vi "KundtsTube.vi"() -> ()   [LabVIEW 2015]
uses:
  <vilib>/imath/engines/lvmath2/RunTimeEngine/Managers/WorkSpace/UID Generator.vi
  <vilib>/imath/engines/lvmath2/RunTimeEngine/RunTimeType/NIMS_RunTimeType_From StrictType (excl LVString).vi
  <instcachedir>/0/NIMS_RunTimeType_From StrictType (excl LVString)_EB1C38A9BC5048DA9ABDA8F781E54D21.lvgen/NIMS_RunTimeType_From StrictType (excl LVString)_EB1C38A9BC5048DA9ABDA8F781E54D21_000.vi
  <vilib>/imath/engines/lvmath2/RunTimeEngine/LocalVariableDefStatement/MC_LocalVariableDefStatement_Display.vi
  <vilib>/imath/engines/lvmath2/RunTimeEngine/Managers/SymbolTable/Clear UID.vi
  <vilib>/imath/engines/lvmath2/RunTimeEngine/NodeEndStatement/NIMS_NodeEndStatement_Output.vi
  <instcachedir>/0/NIMS_NodeEndStatement_Output_53EC0D466D134D7ABD903AC30B43404B.lvgen/NIMS_NodeEndStatement_Output_53EC0D466D134D7ABD903AC30B43404B_009.vi
  <vilib>/imath/engines/lvmath2/RunTimeEngine/ErrorHandling/NIMS_Finalize Error.vi
  <vilib>/imath/engines/lvmath2/RunTimeEngine/Managers/SymbolTable/NIMS_WorkSpace.lvlib
panel:
  out "Gain vs Frequency":dbl[](graph)
  in  "?":enum32{"Single", "Sweep"}(tab)
  in  "Frequency":dbl
  in  "Dwell time, sec":u32
  out "Output":cluster{"RMS":dbl, "Frequency ":dbl}
  in  "?":bool
  in  "Amplitude":dbl
  in  "?":T1
  in  "Sampling Rate (Hz)":dbl
  in  "# of Samples":dbl
  out "Waveform":dbl[](graph)
  # "This will sweep from min to max, pausing by the dwell time after each increment"
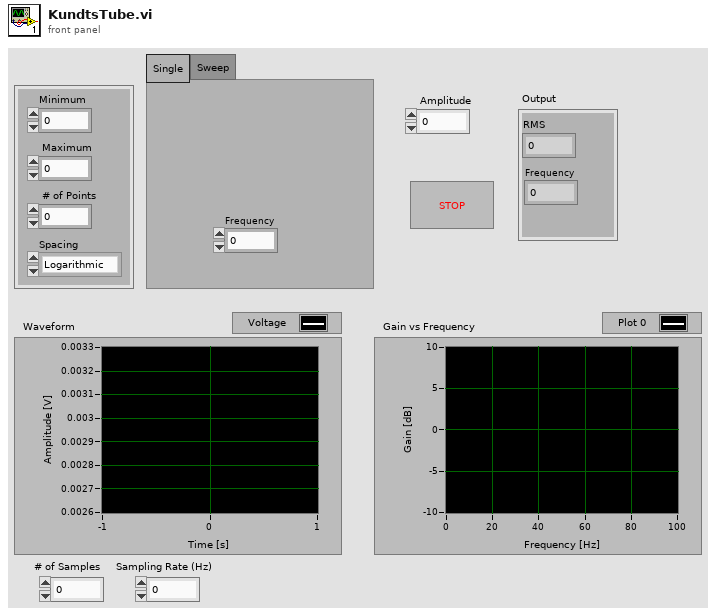
[diagram p1: front panel]
types:
  T1 = cluster{"Minimum":dbl, " Maximum":dbl, "Spacing":enum16{"Logarithmic", "Linear"}, " # of Points":dbl}
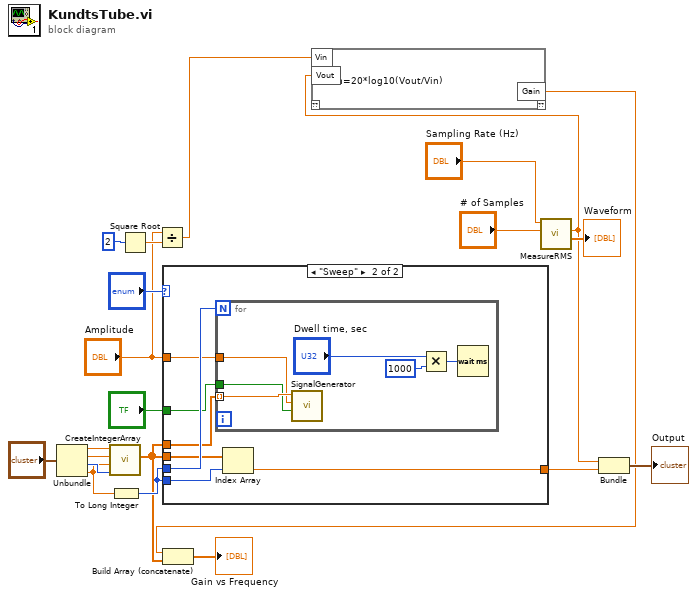
[diagram p0: block diagram]
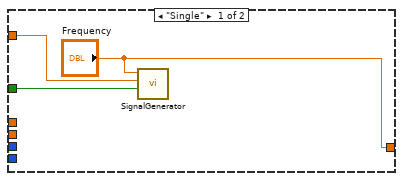
[diagram p2: hidden frame]
diagram:
  n1 = Unbundle("?") -> ("Minimum"=w17:dbl, "Maximum"=w16:dbl, "Spacing"=w15:enum16{"Logarithmic", "Linear"}, "# of Points"=w13:dbl)
  n2 = call "CreateIntegerArray.vi"("Enum"=w15, "# of Points"=w13, "Maximum"=w16, "Minimum"=w17) -> ("Array"=w1:dbl[])  [unwired: 7 in]
  n3 = To Long Integer(number=w13) -> (32bit integer=w2:i32)
  n4 = Square Root(x=2) -> (sqrt(x)=w8:dbl)
  n5 = Divide(x="Amplitude", y=w8) -> (x/y=w6:dbl)
  n6 = case shown="\"Sweep\"" "?" {
    tunnel: w2 -> [_ w31]
    tunnel: w1 -> [_ w30]
    tunnel: "Amplitude" -> [w24 w29]
    tunnel: "?" -> [w23 w28]
    tunnel: ["Frequency" w25] -> w10
    tunnel: w2 -> [_ w27]
    tunnel: w1 -> [_ w26]
    frame "Single" {
      n7 = call "SignalGenerator.vi"("stop"=w23, "Amplitude"=w24, "Frequency"="Frequency") -> ()  [unwired: 7 in, 1 out]
    }
    frame "Sweep" {
      n8 = for {
        N: w31 -> [_]
        tunnel: w30 -> [w37] mode=indexing
        tunnel: w29 -> [w36]
        tunnel: w28 -> [w35]
        n9 = call "SignalGenerator.vi"("stop"=w35, "Amplitude"=w36, "Frequency"=w37) -> ()  [unwired: 7 in, 1 out]
        n10 = Multiply(x="Dwell time, sec", y=1000) -> (x*y=w32:u32)
        n11 = Wait (ms)(milliseconds to wait=w32) -> ()  [unwired: 1 out]
      }
      n12 = Index Array(array=w26, index=w27) -> (element=w25:dbl)
    }
  }
  n13 = call "MeasureRMS.vi"("# of Samples"="# of Samples", "Sampling Rate (Hz)"="Sampling Rate (Hz)") -> ("Waveform Graph"=→"Waveform":dbl[], "RMS"=w5:dbl)  [unwired: 8 in]
  n14 = mathscript code="Gain=20*log10(Vout/Vin)"("Vin"=w6, "Vout"=w5) -> ("Gain"=w4:cdb)  [unwired: 1 in, 1 out]
  n15 = Build Array (concatenate)(w4, w1) -> (→"Gain vs Frequency":cdb[])
  n16 = Bundle("RMS"=w5, "Numeric"=w10) -> (→"Output":cluster{"RMS":dbl, "Numeric":dbl})  [unwired: 1 in]
